vi "Teleop.vi"(10 "Match Info":T1={"Autonomous Elapsed Seconds"=0.0, "TeleOp Elapsed Seconds"=0.0, "Disabled Elapsed Seconds"=0.0, "Visited Autonomous"=FALSE, "Visited TeleOp"=FALSE, "Visited Disabled"=FALSE, "Autonomous Settings"={"Autonomous Style"=enum."Independent", "VI Refnum"=refnum}}, 11 "Call Context":T2) -> ()   [LabVIEW 2019]
doc: "This VI is called for each TeleOp packet received from the DS where the robot is not disabled. It is often used to read from the joysticks and update I/O or to update setpoints for timed control loops. It should complete and return within 20 milliseconds or it may miss DS packets."
uses:
  <vilib>/Rock Robotics/WPI/DriverStation/WPI_DriverStationDerivedRobotMode.ctl
  <vilib>/Rock Robotics/WPI/DriverStation/WPI_DriverStationMatch Info.ctl
  <vilib>/Rock Robotics/WPI/Utilities/WPI_GetSetVariantRefNum.vi
  Robot Global Data.vi
  <vilib>/Rock Robotics/Network Tables/NT Write Number.vi
panel:
  # "Click here to set min"
  # "Click here to set max"
  # "Click here to set min"
  # "Click here to set max"
  # "Click here to set min"
  # "Click here to set max"
  # "Click here to set min"
  # "Click here to set max"
  # "Click here to set min"
  # "Click here to set max"
  # "Click here to set min"
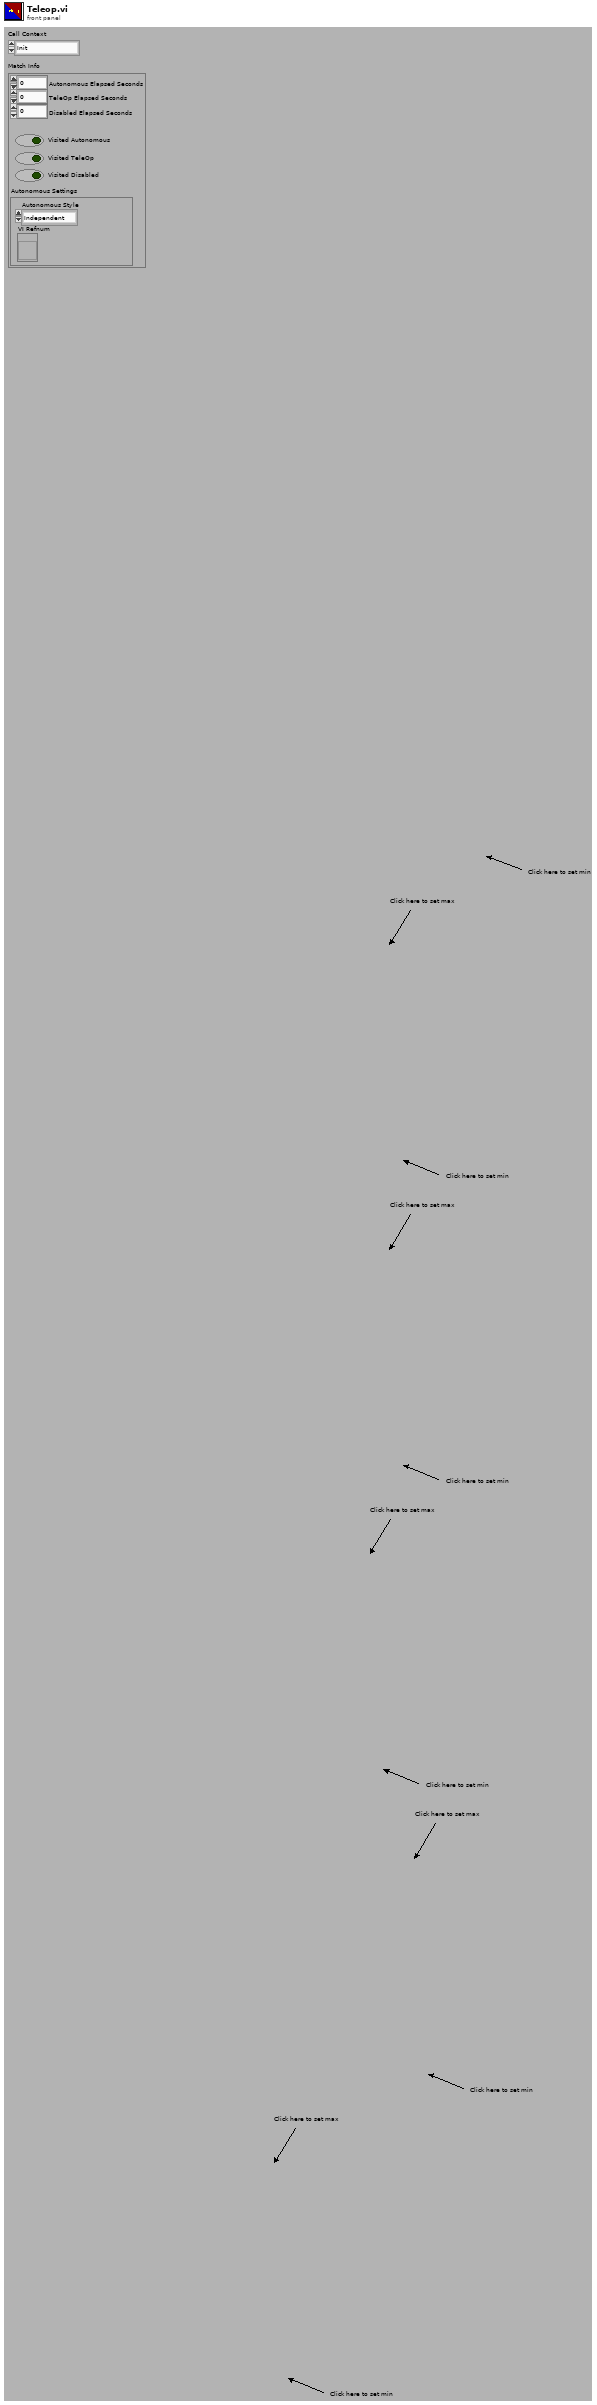
[diagram p1: front panel]
types:
  T1 = typedef "WPI_DriverStationMatch Info.ctl" = cluster{"Autonomous Elapsed Seconds":dbl, "TeleOp Elapsed Seconds":dbl, "Disabled Elapsed Seconds":dbl, "Visited Autonomous":bool, "Visited TeleOp":bool, "Visited Disabled":bool, "Autonomous Settings":cluster{"Autonomous Style":enum16{"Iterative", "Independent"}, "VI Refnum":refnum<vi>}}
  T2 = typedef "WPI_DriverStationDerivedRobotMode.ctl" = enum16{"Init", "Execute", "Stop"}
  T3 = typedef "WPI_JoystickDevRef.ctl" = cluster{"Device":T4}
  T4 = typedef "WPI_JoystickDeviceEnum.ctl" = enum16{"USB 0", "USB 1", "USB 2", "USB 3", "USB 4", "USB 5"}
  T5 = typedef "WPI_RobotDriveDevRef.ctl" = cluster{"DevStatus":errorcluster, "Motors[]":T6[], "Square Inputs":bool, "Max Output":dbl}
  T6 = typedef "WPI_MotorControlDeviceRef.ctl" = cluster{"DeviceStatus":errorcluster, "Type":T7, "PWM":cluster{"PWM Channel":T8, "DeadBand":T9}, "CAN":cluster{"Device Number":u8, "SetOutput VI Ref":variant, "GetOutput VI Ref":variant, "Enable VI Ref":variant, "Disable VI Ref":variant, "Data":variant}, "Invert":bool, "DIO PWM":cluster{"PWM \"Enable\" Channel":T8, "DIOChannel":T10, "PWM Rate":dbl}}
  T7 = typedef "WPI_MotorControlType.ctl" = enum16{"PWM", "CAN", "DIO PWM"}
  T8 = typedef "FPGA_DIOPWMChannel.ctl" = enum8{"PWM 0", "PWM 1", "PWM 2", "PWM 3", "PWM 4", "PWM 5", "PWM 6", "PWM 7", "PWM 8", "PWM 9", "PWM MXP 0", "PWM MXP 1", "PWM MXP 2", "PWM MXP 3", "PWM MXP 4", "PWM MXP 5", "PWM MXP 6", "PWM MXP 7", "PWM MXP 8", "PWM MXP 9", "Invalid"}
  T9 = typedef "WPI_PWMDeadband.ctl" = cluster{"Name":string, "maxPositivePwm":i32, "minPositivePwm":i32, "centerPwm":i32, "maxNegativePwm":i32, "minNegativePwm":i32, "angularRange":u16}
  T10 = typedef "FPGA_DIOChannel.ctl" = enum8{"DIO 0", "DIO 1", "DIO 2", "DIO 3", "DIO 4", "DIO 5", "DIO 6", "DIO 7", "DIO 8", "DIO 9", "DIO MXP 0", "DIO MXP 1", "DIO MXP 2", "DIO MXP 3", "DIO MXP 4", "DIO MXP 5", "DIO MXP 6", "DIO MXP 7", "DIO MXP 8", "DIO MXP 9", "DIO MXP 10", "DIO MXP 11", "DIO MXP 12", "DIO MXP 13", "DIO MXP 14", "DIO MXP 15", "SPI Port CS1", "SPI Port CS2", "SPI Port CS3", "SPI Port MISO", "SPI Port MOSI", "Invalid"}
  T11 = cluster{"JoystickDevRef":T3, "RobotDriveDevRef":T5}
  T12 = typedef "WPI_ServoDeviceRef.ctl" = cluster{"DeviceStatus":errorcluster, "PWM Channel":T8, "DeadBand":T9}
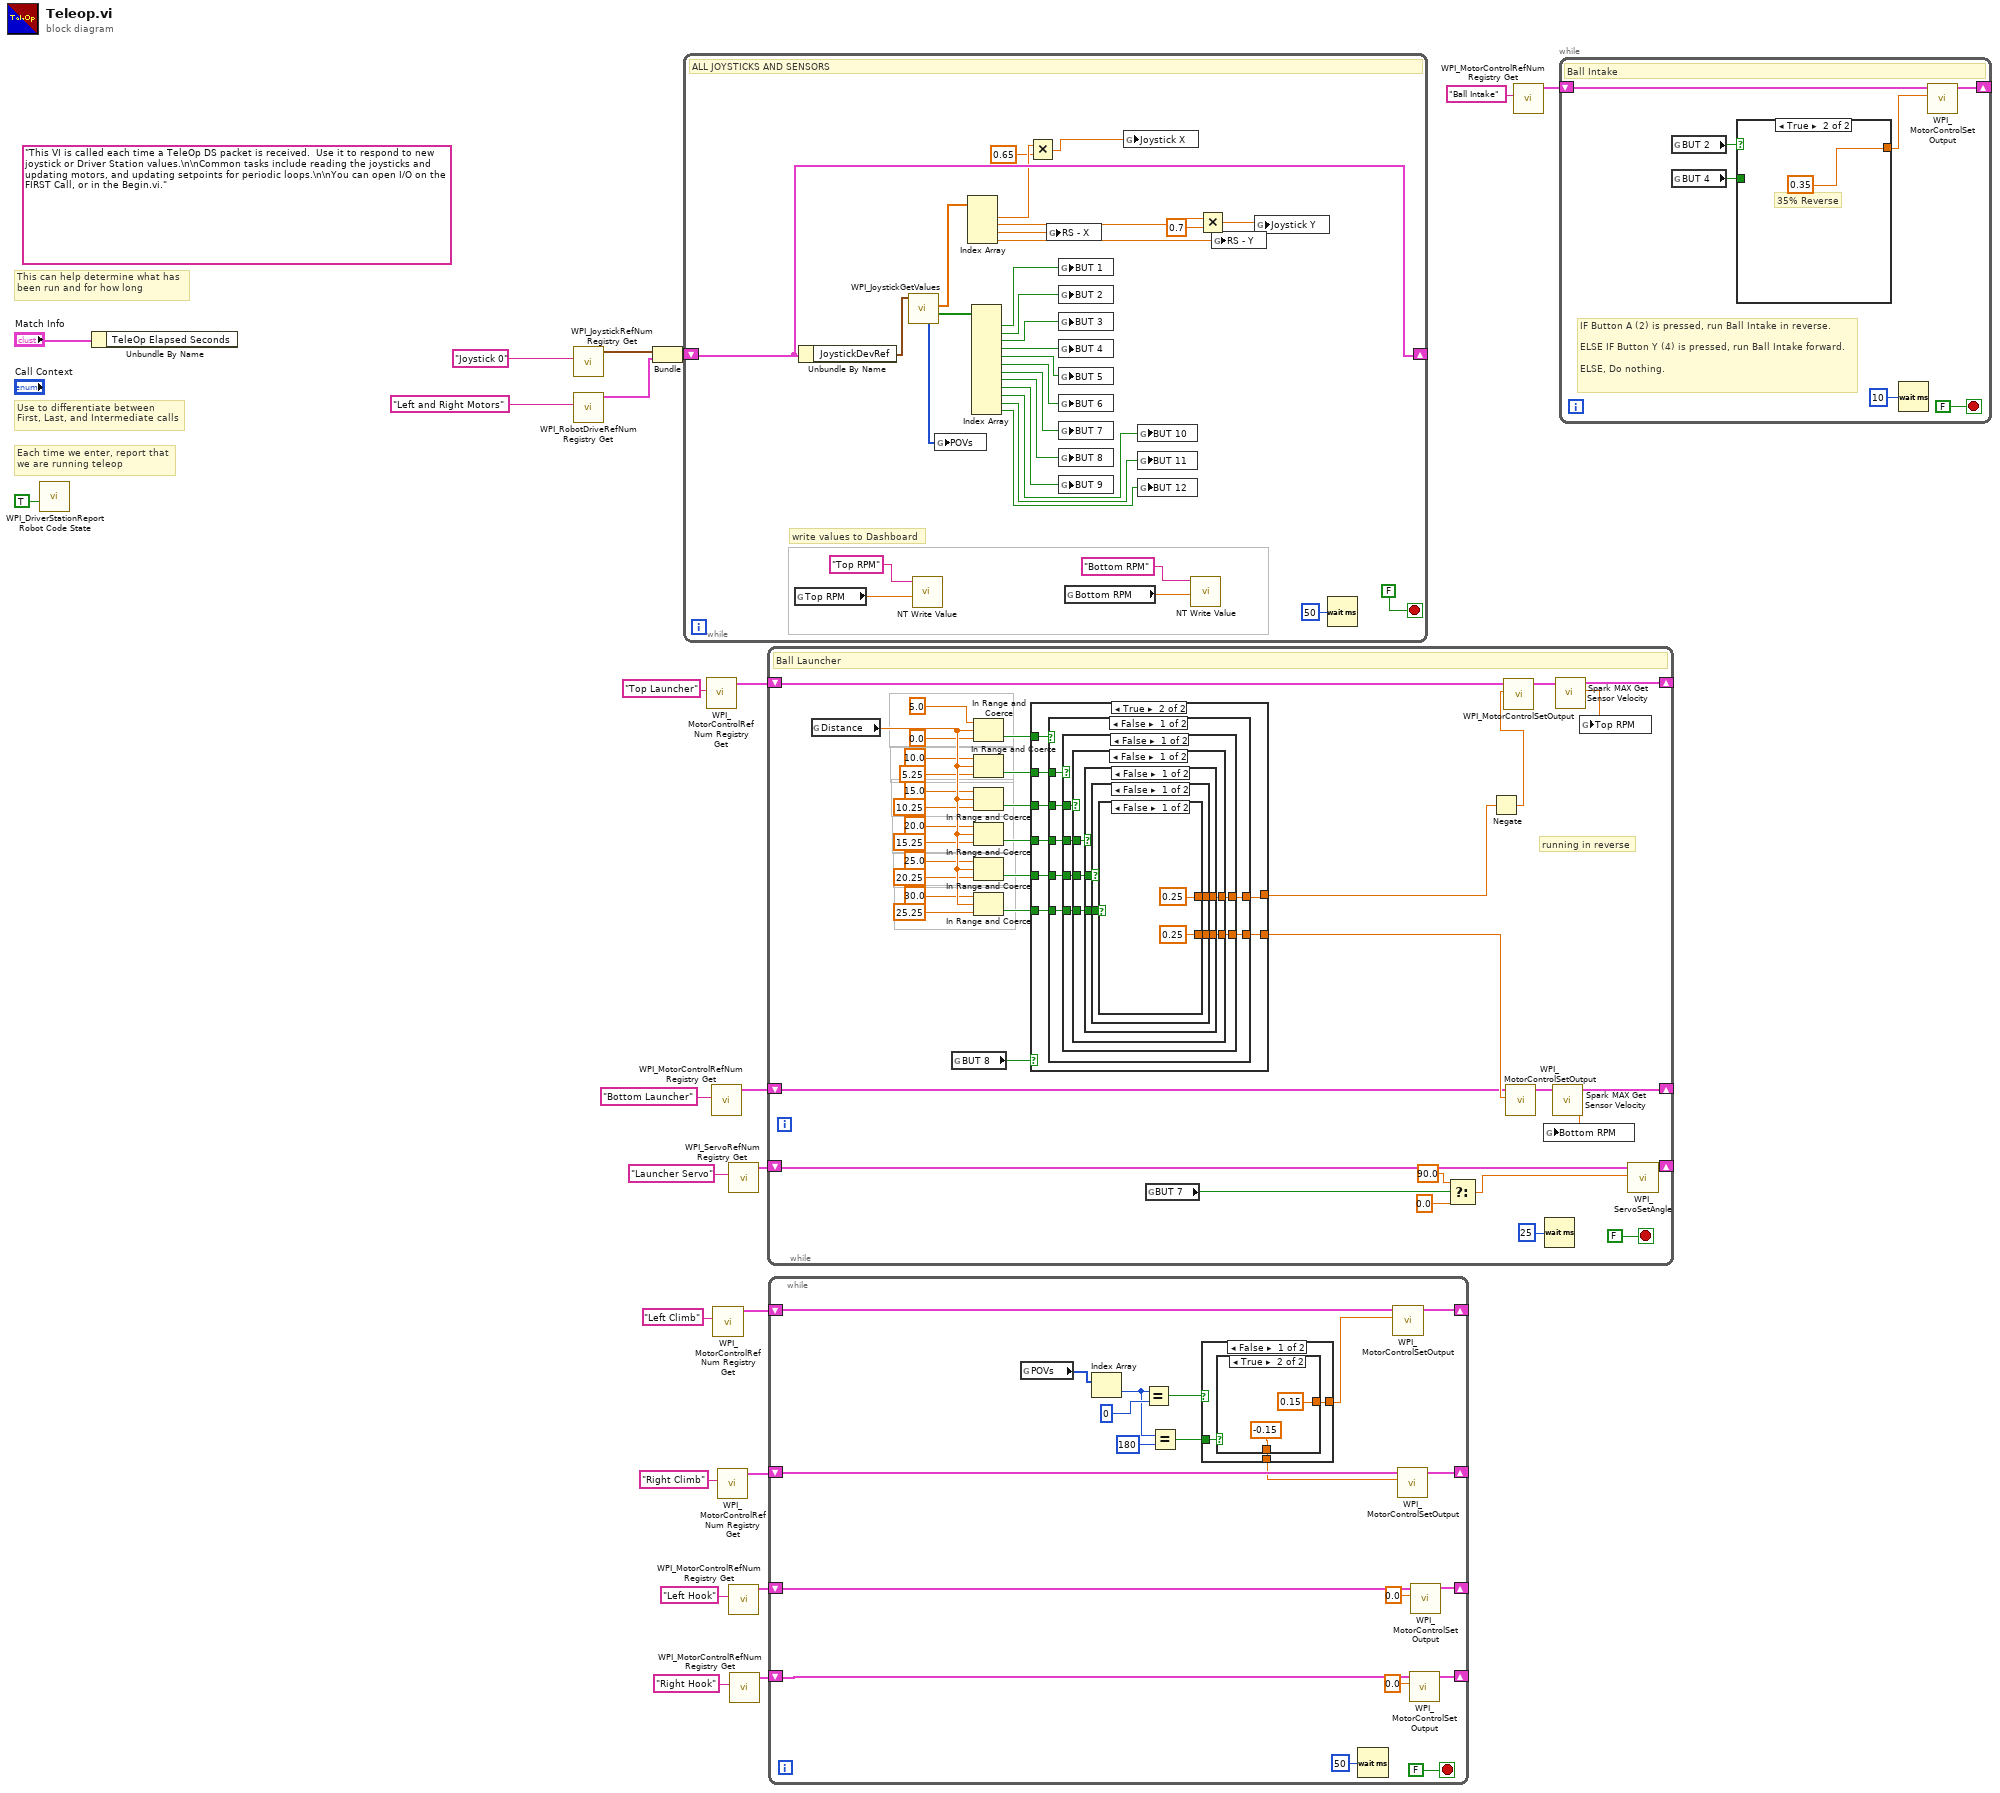
[diagram p0: block diagram]
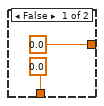
[diagram p2: hidden frame]
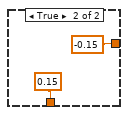
[diagram p3: hidden frame]
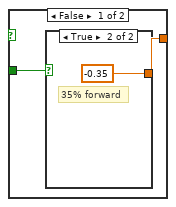
[diagram p4: hidden frame]
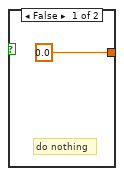
[diagram p5: hidden frame]
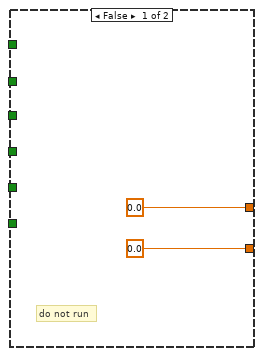
[diagram p6: hidden frame]
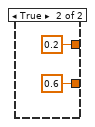
[diagram p7: hidden frame]
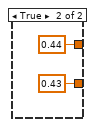
[diagram p8: hidden frame]
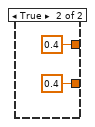
[diagram p9: hidden frame]
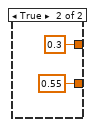
[diagram p10: hidden frame]
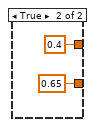
[diagram p11: hidden frame]
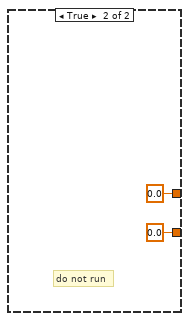
[diagram p12: hidden frame]
diagram:
  (unwired) "This VI is called each time a TeleOp DS packet is received.  Use it to respond to new joystick or Driver Station values.\n\nCommon tasks include reading the joysticks and updating motors, and updating setpoints for periodic loops.\n\nYou can open I/O on the FIRST Call, or in the Begin.vi."
  # "Each time we enter, report that\nwe are running teleop"
  # "Use to differentiate between\nFirst, Last, and Intermediate calls"
  # "This can help determine what has\nbeen run and for how long"
  n1 = call <vilib>:"WPI_DriverStationReport Robot Code State.vi"("TeleOp"=TRUE ("Autonomous")) -> ()  [unwired: 10 in, 1 out]
  n2 = Unbundle By Name("Match Info") -> ()  [unwired: 1 out]
  n3 = call <vilib>:"WPI_JoystickRefNum Registry Get.vi"("refnum name"="Joystick 0") -> ("JoystickDevRef"=w19:T3)  [unwired: 1 in, 9 out]
  n4 = call <vilib>:"WPI_RobotDriveRefNum Registry Get.vi"("refnum name"="Left and Right Motors") -> ("RobotDriveDevRef"=w18:T5)  [unwired: 1 in, 9 out]
  n5 = Bundle("JoystickDevRef"=w19, "RobotDriveDevRef"=w18) -> (w17:T11)  [unwired: 1 out]
  n6 = while {
    shift-right: [w39] -> _
    shift-left: w17 -> [w39]
    stop <- FALSE stop-if-true
    # "write values to Dashboard"
    # "ALL JOYSTICKS AND SENSORS"
    n7 = global read "Robot Global Data.vi" "Top RPM"() -> (w34:dbl)
    n8 = Unbundle By Name(w39) -> ("JoystickDevRef"=w53:T3)
    n9 = call <vilib>:"WPI_JoystickGetValues.vi"("JoystickDevRef"=w53) -> ("Buttons"=w52:bool[], "Axes"=w38:dbl[], "POVs"=w30:i16[])  [unwired: 6 in, 2 out]
    n10 = call-poly <vilib>:"NT Write Value.vi"("Numeric"=w34, "Name"="Top RPM") -> ()  [unwired: 9 in, 1 out]
    n11 = global write "Robot Global Data.vi" "POVs"(w30) -> ()
    n12 = Index Array(array=w38) -> (element #1=w27:dbl, element #2=w29:dbl, element #3=w31:dbl, element #4=w37:dbl)  [unwired: 4 in]
    n13 = Index Array(array=w52) -> (element #1=w51:bool, element #2=w50:bool, element #3=w49:bool, element #4=w48:bool, element #5=w47:bool, element #6=w46:bool, element #7=w45:bool, element #8=w44:bool, element #9=w43:bool, element #10=w42:bool, element #11=w41:bool, element #12=w40:bool)  [unwired: 12 in]
    n14 = Multiply(x=w27, y=0.65) -> (x*y=w28:dbl)
    n15 = global write "Robot Global Data.vi" "RS - X"(w31) -> ()
    n16 = global write "Robot Global Data.vi" "BUT 1"(w51) -> ()
    n17 = global write "Robot Global Data.vi" "BUT 2"(w50) -> ()
    n18 = global write "Robot Global Data.vi" "BUT 3"(w49) -> ()
    n19 = global write "Robot Global Data.vi" "BUT 4"(w48) -> ()
    n20 = global write "Robot Global Data.vi" "BUT 5"(w47) -> ()
    n21 = global write "Robot Global Data.vi" "BUT 6"(w46) -> ()
    n22 = global write "Robot Global Data.vi" "BUT 7"(w45) -> ()
    n23 = global write "Robot Global Data.vi" "BUT 8"(w44) -> ()
    n24 = global write "Robot Global Data.vi" "BUT 9"(w43) -> ()
    n25 = global read "Robot Global Data.vi" "Bottom RPM"() -> (w32:dbl)
    n26 = global write "Robot Global Data.vi" "Joystick X"(w28) -> ()
    n27 = global write "Robot Global Data.vi" "BUT 10"(w42) -> ()
    n28 = global write "Robot Global Data.vi" "BUT 11"(w41) -> ()
    n29 = global write "Robot Global Data.vi" "BUT 12"(w40) -> ()
    n30 = call-poly <vilib>:"NT Write Value.vi"("Numeric"=w32, "Name"="Bottom RPM") -> ()  [unwired: 9 in, 1 out]
    n31 = Multiply(x=w29, y=0.7) -> (x*y=w25:dbl)
    n32 = global write "Robot Global Data.vi" "RS - Y"(w37) -> ()
    n33 = global write "Robot Global Data.vi" "Joystick Y"(w25) -> ()
    n34 = Wait (ms)(milliseconds to wait=u32 50) -> ()  [unwired: 1 out]
  }
  n35 = call <vilib>:"WPI_MotorControlRefNum Registry Get.vi"("refnum name"="Top Launcher") -> ("MotorControlDevRef"=w13:T6)  [unwired: 9 in, 1 out]
  n36 = call <vilib>:"WPI_MotorControlRefNum Registry Get.vi"("refnum name"="Bottom Launcher") -> ("MotorControlDevRef"=w15:T6)  [unwired: 9 in, 1 out]
  n37 = call <vilib>:"WPI_MotorControlRefNum Registry Get.vi"("refnum name"="Left Climb") -> ("MotorControlDevRef"=w7:T6)  [unwired: 9 in, 1 out]
  n38 = call <vilib>:"WPI_MotorControlRefNum Registry Get.vi"("refnum name"="Right Climb") -> ("MotorControlDevRef"=w6:T6)  [unwired: 9 in, 1 out]
  n39 = call <vilib>:"WPI_ServoRefNum Registry Get.vi"("refnum name"="Launcher Servo") -> ("ServoDeviceRef"=w11:T12)  [unwired: 9 in, 1 out]
  n40 = call <vilib>:"WPI_MotorControlRefNum Registry Get.vi"("refnum name"="Left Hook") -> ("MotorControlDevRef"=w2:T6)  [unwired: 9 in, 1 out]
  n41 = call <vilib>:"WPI_MotorControlRefNum Registry Get.vi"("refnum name"="Right Hook") -> ("MotorControlDevRef"=w3:T6)  [unwired: 9 in, 1 out]
  n42 = while {
    shift-right: [w63] -> _
    shift-left: w15 -> [w64]
    shift-right: [w61] -> _
    shift-left: w13 -> [w62]
    shift-right: [w60] -> _
    shift-left: w11 -> [w55]
    stop <- FALSE stop-if-true
    # "running in reverse"
    # "Ball Launcher"
    n43 = global read "Robot Global Data.vi" "Distance"() -> (w93:dbl)
    n44 = global read "Robot Global Data.vi" "BUT 8"() -> (w71:bool)
    n45 = In Range and Coerce(upper limit=5.0, x=w93, lower limit=0.0) -> (In Range?=w90:bool)  [unwired: 1 out]
    n46 = In Range and Coerce(upper limit=10.0, x=w93, lower limit=5.25) -> (In Range?=w89:bool)  [unwired: 1 out]
    n47 = In Range and Coerce(upper limit=15.0, x=w93, lower limit=10.25) -> (In Range?=w73:bool)  [unwired: 1 out]
    n48 = In Range and Coerce(upper limit=20.0, x=w93, lower limit=15.25) -> (In Range?=w74:bool)  [unwired: 1 out]
    n49 = In Range and Coerce(upper limit=25.0, x=w93, lower limit=20.25) -> (In Range?=w75:bool)  [unwired: 1 out]
    n50 = In Range and Coerce(upper limit=30.0, x=w93, lower limit=25.25) -> (In Range?=w76:bool)  [unwired: 1 out]
    n51 = case shown="True" w71 {
      tunnel: [0.0 ("Output") w97] -> w92
      tunnel: [0.0 ("Output") w96] -> w72
      tunnel: w90 -> [_ w103]
      tunnel: w73 -> [_ w101]
      tunnel: w74 -> [_ w100]
      tunnel: w75 -> [_ w99]
      tunnel: w76 -> [_ w98]
      tunnel: w89 -> [_ w102]
      frame False {
        # "do not run"
      }
      frame True {
        n52 = case shown="False" w103 {
          tunnel: w102 -> [w110 _]
          tunnel: w101 -> [w109 _]
          tunnel: w100 -> [w108 _]
          tunnel: w99 -> [w107 _]
          tunnel: w98 -> [w106 _]
          tunnel: [w105 0.0 ("Output")] -> w97
          tunnel: [w104 0.0 ("Output")] -> w96
          frame False {
            n53 = case shown="False" w110 {
              tunnel: w109 -> [w116 _]
              tunnel: w108 -> [w115 _]
              tunnel: w107 -> [w114 _]
              tunnel: w106 -> [w113 _]
              tunnel: [w112 0.4 ("Output")] -> w105
              tunnel: [w111 0.65 ("Output")] -> w104
              frame False {
                n54 = case shown="False" w116 {
                  tunnel: w115 -> [w121 _]
                  tunnel: w114 -> [w120 _]
                  tunnel: w113 -> [w119 _]
                  tunnel: [w118 0.3 ("Output")] -> w112
                  tunnel: [w117 0.55 ("Output")] -> w111
                  frame False {
                    n55 = case shown="False" w121 {
                      tunnel: w120 -> [w125 _]
                      tunnel: w119 -> [w124 _]
                      tunnel: [w123 0.4 ("Output")] -> w118
                      tunnel: [w122 0.4 ("Output")] -> w117
                      frame False {
                        n56 = case shown="False" w125 {
                          tunnel: w124 -> [w128 _]
                          tunnel: [w127 0.44 ("Output")] -> w123
                          tunnel: [w126 0.43 ("Output")] -> w122
                          frame False {
                            n57 = case shown="False" w128 {
                              tunnel: [0.25 ("Output") 0.2 ("Output")] -> w127
                              tunnel: [0.25 ("Output") 0.6 ("Output")] -> w126
                              frame False {
                              }
                              frame True {
                              }
                            }
                          }
                          frame True {
                          }
                        }
                      }
                      frame True {
                      }
                    }
                  }
                  frame True {
                  }
                }
              }
              frame True {
              }
            }
          }
          frame True {
            # "do not run"
          }
        }
      }
    }
    n58 = global read "Robot Global Data.vi" "BUT 7"() -> (w59:bool)
    n59 = Select(t=90.0, s=w59, f=0.0) -> (s? t:f=w56:dbl)
    n60 = Negate(x=w92) -> (-x=w91:dbl)
    n61 = call <vilib>:"WPI_MotorControlSetOutput.vi"("Output"=w91, "MotorControlDevRef"=w62) -> ("MotorControlDevRef"=w69:T6)  [unwired: 7 in, 2 out]
    n62 = call <vilib>:"WPI_MotorControlSetOutput.vi"("Output"=w72, "MotorControlDevRef"=w64) -> ("MotorControlDevRef"=w70:T6)  [unwired: 7 in, 2 out]
    n63 = Wait (ms)(milliseconds to wait=u32 25) -> ()  [unwired: 1 out]
    n64 = call <vilib>:"Spark MAX Get Sensor Velocity.vi"("MotorControlDevRef in"=w70) -> ("Sensor Velocity"=w68:dbl, "MotorControlDevRef out"=w63:T6)  [unwired: 7 in, 2 out]
    n65 = global write "Robot Global Data.vi" "Bottom RPM"(w68) -> ()
    n66 = call <vilib>:"Spark MAX Get Sensor Velocity.vi"("MotorControlDevRef in"=w69) -> ("Sensor Velocity"=w67:dbl, "MotorControlDevRef out"=w61:T6)  [unwired: 7 in, 2 out]
    n67 = global write "Robot Global Data.vi" "Top RPM"(w67) -> ()
    n68 = call <vilib>:"WPI_ServoSetAngle.vi"("Angle"=w56, "ServoDeviceRef"=w55) -> ("ServoDeviceRef"=w60:T12)  [unwired: 8 in, 1 out]
  }
  n69 = while {
    shift-right: [w161] -> _
    shift-left: w7 -> [w160]
    shift-right: [w158] -> _
    shift-left: w6 -> [w159]
    shift-right: [w147] -> _
    shift-left: w3 -> [w148]
    shift-right: [w145] -> _
    shift-left: w2 -> [w146]
    stop <- FALSE stop-if-true
    n70 = global read "Robot Global Data.vi" "POVs"() -> (w155:i16[])
    n71 = Index Array(array=w155) -> (element=w153:i16)  [unwired: 1 in]
    n72 = Equal?(x=w153, y=i16 0) -> (x = y?=w151:bool)
    n73 = Equal?(x=w153, y=i16 180) -> (x = y?=w150:bool)
    n74 = case shown="False" w151 {
      tunnel: [w165 -0.15 ("Output")] -> w157
      tunnel: [w164 0.15 ("Output")] -> w156
      tunnel: w150 -> [w163 _]
      frame False {
        n75 = case shown="True" w163 {
          tunnel: [0.0 ("Output") 0.15 ("Output")] -> w165
          tunnel: [0.0 ("Output") -0.15 ("Output")] -> w164
          frame False {
          }
          frame True {
          }
        }
      }
      frame True {
      }
    }
    n76 = Wait (ms)(milliseconds to wait=u32 50) -> ()  [unwired: 1 out]
    n77 = call <vilib>:"WPI_MotorControlSetOutput.vi"("Output"=w157, "MotorControlDevRef"=w160) -> ("MotorControlDevRef"=w161:T6)  [unwired: 7 in, 2 out]
    n78 = call <vilib>:"WPI_MotorControlSetOutput.vi"("Output"=w156, "MotorControlDevRef"=w159) -> ("MotorControlDevRef"=w158:T6)  [unwired: 7 in, 2 out]
    n79 = call <vilib>:"WPI_MotorControlSetOutput.vi"("Output"=0.0, "MotorControlDevRef"=w148) -> ("MotorControlDevRef"=w147:T6)  [unwired: 7 in, 2 out]
    n80 = call <vilib>:"WPI_MotorControlSetOutput.vi"("Output"=0.0, "MotorControlDevRef"=w146) -> ("MotorControlDevRef"=w145:T6)  [unwired: 7 in, 2 out]
  }
  n81 = call <vilib>:"WPI_MotorControlRefNum Registry Get.vi"("refnum name"="Ball Intake") -> ("MotorControlDevRef"=w9:T6)  [unwired: 9 in, 1 out]
  n82 = while {
    shift-right: [w175] -> _
    shift-left: w9 -> [w176]
    stop <- FALSE stop-if-true
    # "IF Button A (2) is pressed, run Ball Intake in reverse. \n\nELSE IF Button Y (4) is pressed, run Ball Intake forward.\n\nELSE, Do nothing."
    # "Ball Intake"
    n83 = global read "Robot Global Data.vi" "BUT 2"() -> (w173:bool)
    n84 = global read "Robot Global Data.vi" "BUT 4"() -> (w174:bool)
    n85 = case shown="True" w173 {
      tunnel: [w180 0.35 ("Output")] -> w172
      tunnel: w174 -> [w179 _]
      frame False {
        n86 = case shown="True" w179 {
          tunnel: [0.0 ("Output") -0.35 ("Output")] -> w180
          frame False {
            # "do nothing"
          }
          frame True {
            # "35% forward"
          }
        }
      }
      frame True {
        # "35% Reverse"
      }
    }
    n87 = Wait (ms)(milliseconds to wait=u32 10) -> ()  [unwired: 1 out]
    n88 = call <vilib>:"WPI_MotorControlSetOutput.vi"("Output"=w172, "MotorControlDevRef"=w176) -> ("MotorControlDevRef"=w175:T6)  [unwired: 7 in, 2 out]
  }
